vi "TSM Relay Control Config.vi"(0 "TSM Relay Configuration in":T1 {"SSC Relay with Action"."Relay Action" items=["Open Relay"=20, "Close Relay"=21]}, 7 "Settling Time (s)":dbl, 11 "error in":errorcluster) -> (4 "TSM Relay Configuration out":T1 {"SSC Relay with Action"."Relay Action" items=["Open Relay"=20, "Close Relay"=21]}, 8 "Completed Relay Operations":T4[](array[typedef]) {"Desired State" items=["Open Relay"=20, "Close Relay"=21]}, 15 "error out":errorcluster)   [LabVIEW 2019]
doc: "Performs the actions as specified in the TSM Relay Configuration session."
uses:
  SubVIs/TSM Relay Config.ctl
  <vilib>/NI_TestStand_SemiconductorModule/NI_TestStand_Semiconductor_Module.lvlibp/PinMap/PinQueryContext/MultiplePinMultipleSessionQueryContext/MultiplePinMultipleSessionQueryContext.lvclass
  SSC/SSC Relay.ctl
  <instrlib>/niSwitch/niSwitch.llb/niSwitch Relay Action.ctl
  SubVIs/TSM Relay Completed Operations.ctl
  SSC/Single SSC Relay NI-Switch Control.vi
  SSC/Single SSC Relay Fill Additional Error info.vi
  SSC/SSC Relay Expand Action Array to All Sessions.vi
  <vilib>/Utility/error.llb/Error Cluster From Error Code.vi
  <instrlib>/niSwitch/niSwitch.llb/niSwitch Get Relay Position.vi
  <instrlib>/niSwitch/niSwitch.llb/niSwitch Relay Control.vi
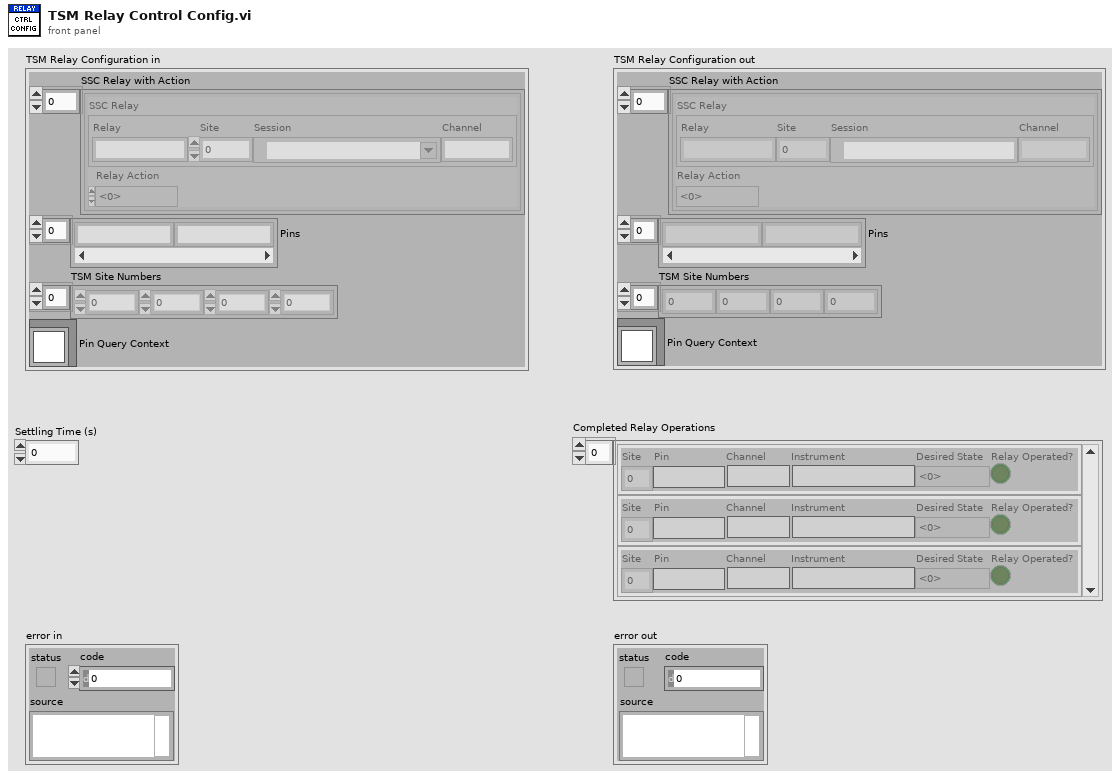
[diagram p1: front panel]
types:
  T1 = typedef "TSM Relay Config.ctl" = cluster{"SSC Relay with Action":cluster{"SSC Relay":T2, "Relay Action":T3}[], "Pins":string[], "TSM Site Numbers":i32[], "Pin Query Context":refnum<class "MultiplePinMultipleSessionQueryContext.lvclass">}
  T2 = typedef "SSC Relay.ctl" = cluster{"Relay":string, "Site":i32, "Session":refnum<k15>, "Channel":string}
  T3 = typedef "niSwitch Relay Action.ctl" = i32
  T4 = typedef "TSM Relay Completed Operations.ctl" = cluster{"Site":i32, "Pin":string, "Channel":string, "Instrument":string, "Desired State":T3, "Relay Operated?":bool}
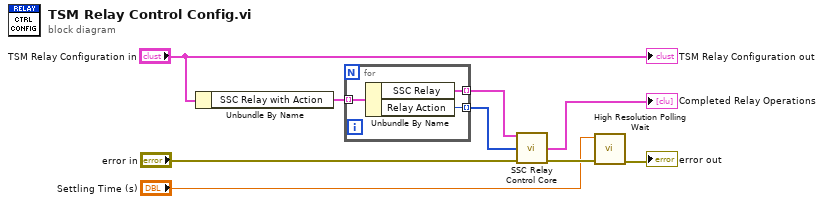
[diagram p0: block diagram]
diagram:
  n1 = Unbundle By Name("TSM Relay Configuration in") -> ("SSC Relay with Action"=w6:cluster{"SSC Relay":T2, "Relay Action":T3}[])
  n2 = for {
    tunnel: [w12] -> w5 mode=indexing
    tunnel: w6 -> [w11] mode=indexing
    tunnel: [w10] -> w4 mode=indexing
    n3 = Unbundle By Name(w11) -> ("SSC Relay"=w10:T2, "Relay Action"=w12:T3)
  }
  n4 = call "SSC Relay Control Core.vi"("SSC Relay in"=w4, "Relay Commands"=w5, "error in"="error in") -> ("Completed Relay Operations"=→"Completed Relay Operations":T4[], "error out"=w7:errorcluster)  [unwired: 10 in, 1 out]
  n5 = call <vilib>:"High Resolution Polling Wait.vi"("error in (no error)"=w7, "seconds to wait"="Settling Time (s)") -> ("error out"=→"error out":errorcluster)  [unwired: 9 in]
  "TSM Relay Configuration out" <- "TSM Relay Configuration in"
